vi "FABR-Init SCL.vi"(0 "Sequence":T2={"Freq"={"Expression"="", "Step"=80}, "Level"={"Start (dB)"=20, "Stop (dB)"=80, "Step (dB)"=5}, "Order"=enum."Interleaved"} {"Level"."Start (dB)" step=5}, 5 "Frequency":dbl[](array[numeric]), 7 "Ceiling":dbl[](array[numeric]), 9 "Order":i32[](array[numeric]), 11 "error in (no error)":errorcluster) -> (6 "SCL":cluster{T1[]}[](array[cluster]), 14 "Level":dbl[](array[numeric]), 15 "error out":errorcluster)   [LabVIEW 2020]
uses:
  Typedefs/FABR-Sequence.ctl
  Typedefs/FABR-Order.ctl
  Typedefs/FABR-Stimulus Condition.ctl
  epl-vi-lib/Utility VIs/Math VIs/LinSpace (start-stop-step).vi
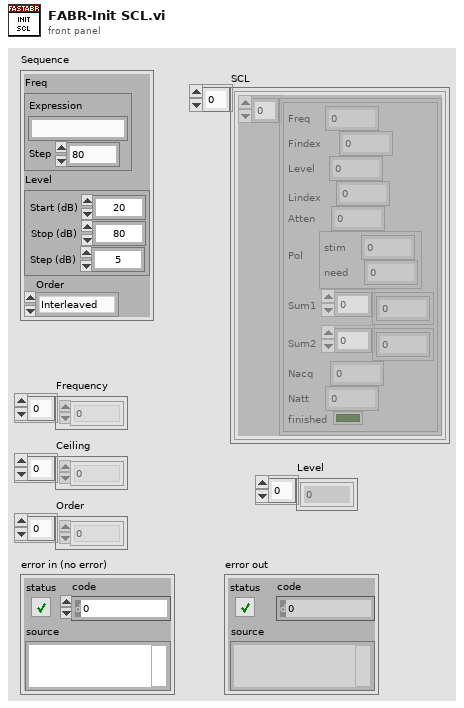
[diagram p1: front panel]
types:
  T1 = typedef "FABR-Stimulus Condition.ctl" = cluster{"Freq":dbl, "Findex":i32, "Level":dbl, "Lindex":i32, "Atten":dbl, "Pol":cluster{"stim":i32, "need":i32}, "Sum1":dbl[], "Sum2":dbl[], "Nacq":i32, "Natt":i32, "finished":bool}
  T2 = typedef "FABR-Sequence.ctl" = cluster{"Freq":cluster{"Expression":string, "Step":i32}, "Level":cluster{"Start (dB)":i32, "Stop (dB)":i32, "Step (dB)":i32}, "Order":T3}
  T3 = typedef "FABR-Order.ctl" = enum16{"Interleaved"}
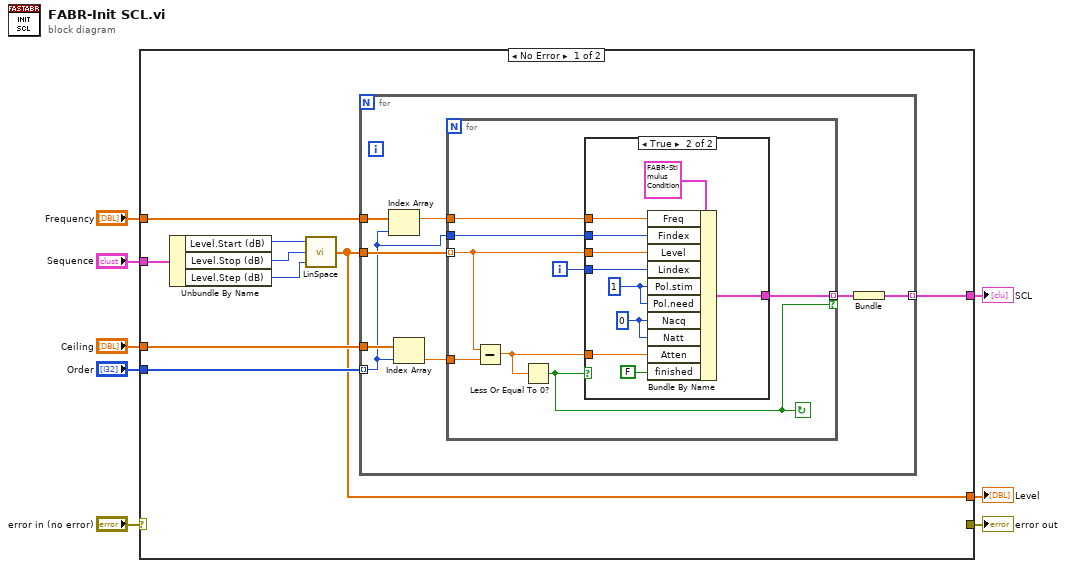
[diagram p0: block diagram]
diagram:
  n1 = case shown="No Error" "error in (no error)" {
    selector: "error in (no error)" -> [_ w44]
    tunnel: "Sequence" -> [w17 _]
    tunnel: [_ w44] -> w6
    tunnel: "Frequency" -> [w13 _]
    tunnel: [w12 _] -> w2
    tunnel: "Order" -> [w11 _]
    tunnel: "Ceiling" -> [w10 _]
    tunnel: [w9 _] -> w1
    frame No Error {
      n2 = Unbundle By Name(w17) -> ("Level.Start (dB)"=w16:i32, "Level.Stop (dB)"=w15:i32, "Level.Step (dB)"=w14:i32)
      n3 = call-poly "LinSpace.vi"("Step"=w14, "Stop"=w15, "Start"=w16) -> ("Array"=w9:dbl[])  [unwired: 1 in, 1 out]
      n4 = for {
        tunnel: w13 -> [w25]
        tunnel: w9 -> [w24]
        tunnel: [w22] -> w12 mode=indexing
        tunnel: w11 -> [w19] mode=indexing
        tunnel: w10 -> [w20]
        n5 = Index Array(array=w25, index=w19) -> (element=w21:dbl)
        n6 = Index Array(array=w20, index=w19) -> (element=w18:dbl)
        n7 = for {
          tunnel: w21 -> [w33]
          tunnel: w19 -> [w32]
          tunnel: [w31] -> w23 mode=indexing if=w27
          tunnel: w24 -> [w29] mode=indexing
          tunnel: w18 -> [w28]
          i -> [w30]
          stop <- w27 continue-if-true
          n8 = Subtract(x=w29, y=w28) -> (x-y=w26:dbl)
          n9 = Less Or Equal To 0?(x=w26) -> (x <= 0?=w27:bool)
          n10 = case shown="True" w27 {
            tunnel: w33 -> [_ w42]
            tunnel: w32 -> [_ w41]
            tunnel: w29 -> [_ w40]
            tunnel: [_ w37] -> w31
            tunnel: w30 -> [_ w35]
            tunnel: w26 -> [_ w34]
            frame False {
            }
            frame True {
              w39 = 0 ("Nacq")
              w36 = 1 ("Pol")
              n11 = Bundle By Name(cluster=T1 {"Freq"=0.0, "Findex"=0, "Level"=0.0, "Lindex"=0, "Atten"=0.0, "Pol"={"stim"=0, "need"=0}, "Sum1"=[], "Sum2"=[], "Nacq"=0, "Natt"=0, "finished"=FALSE} ("SC"), "Freq"=w42, "Findex"=w41, "Level"=w40, "Lindex"=w35, "Pol.stim"=w36, "Pol.need"=w36, "Nacq"=w39, "Natt"=w39, "Atten"=w34, "finished"=FALSE) -> (w37:T1)
            }
          }
        }
        n12 = Bundle(w23) -> (w22:cluster{T1[]})  [unwired: 1 in]
      }
    }
    frame Error {
    }
  }
  "error out" <- w6
  "SCL" <- w2
  "Level" <- w1
